vi "Globals.vi"() -> ()   [LabVIEW 2015]
panel:
  in  "exp time":dbl
  in  "nos":dbl
  in  "PIXEL":dbl
  in  "boards":dbl
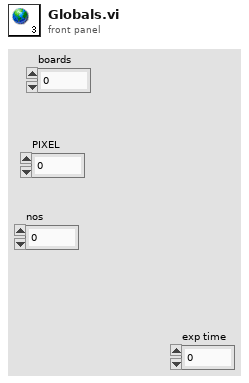
[diagram p1: front panel]
diagram:
